vi "ModbusRdWrCam3.vi"() -> ()   [LabVIEW 2020]
uses:
  <vilib>/userdefined/High Color/IMAQdx.ctl
  <vilib>/Modbus/master/Create Master Instance (TCP).vi
  <vilib>/Modbus/master/Modbus Master.lvclass
  <vilib>/vision/driver/NI_Vision_Acquisition_Software.lvlib
panel:
  in  "Off/On":bool=TRUE
  out "Cam":bool
  in  "Session":T1="cam1"
  out "Image":T2(plugin-control)
  in  "5":i16(slide)=300 min=80 max=520 step=5 scale=80.0..520.0
  in  "4":i16(slide)=310 min=80 max=520 step=5 scale=80.0..520.0
  in  "3":i16(slide)=120 min=80 max=520 step=5 scale=80.0..520.0
  in  "2":i16(slide)=450 min=80 max=520 step=5 scale=80.0..520.0
  in  "1":i16(slide)=380 min=80 max=520 step=5 scale=80.0..520.0
  out "Modbus":bool
  in  "ip":string="192.168.4.1"
  out "Timer":u16=704
  in  "0":i16(slide)=285 min=80 max=520 step=5 scale=80.0..520.0
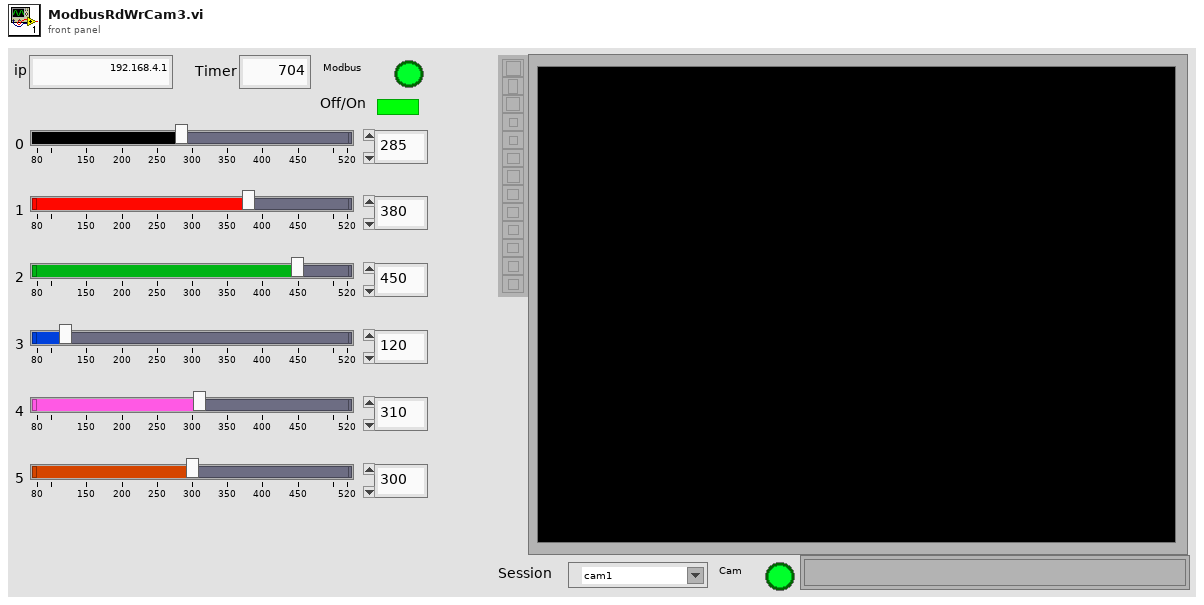
[diagram p1: front panel]
types:
  T1 = typedef "IMAQdx.ctl" = refnum<k21>
  T2 = typedef "IMAQ Image.ctl" = refnum<image>
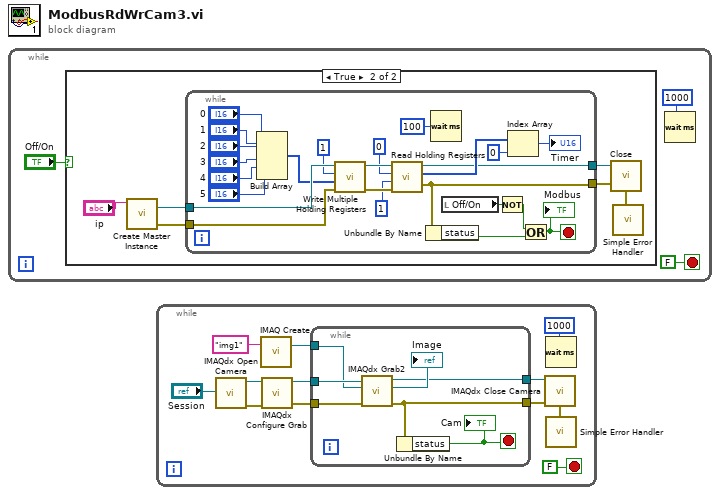
[diagram p0: block diagram]
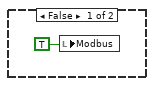
[diagram p2: hidden frame]
diagram:
  n1 = while {
    stop <- FALSE stop-if-true
    n2 = case shown="True" "Off/On" {
      frame False {
        n3 = local write "Modbus"(TRUE) -> ()
      }
      frame True {
        n4 = call-poly <vilib>:"Create Master Instance.vi"("address"="ip") -> ("error out"=w8:errorcluster, "TCP master instance"=w9:refnum<class "Modbus Master.lvclass">)  [unwired: 9 in]
        n5 = while {
          tunnel: w9 -> [w33]
          tunnel: w8 -> [w22]
          tunnel: [w14] -> w7
          tunnel: [w13] -> w6
          stop <- w16 stop-if-true
          n6 = Build Array("0", "1", "2", "3", "4", "5") -> (w32:i16[])
          n7 = call-dynamic "Write Multiple Holding Registers.vi"("error in (no error)"=w22, "holding register values"=w32, "starting address"=u16 1, "Modbus master in"=w33) -> ("error out"=w27:errorcluster, "Modbus master out"=w28:refnum<class "Modbus Master.lvclass">)  [unwired: 6 in]
          n8 = call-dynamic "Read Holding Registers.vi"("error in (no error)"=w27, "number of holding registers"=u16 1, "starting address"=u16 0, "Modbus master in"=w28) -> ("error out"=w13:errorcluster, "register values"=w24:u16[], "Modbus master out"=w14:refnum<class "Modbus Master.lvclass">)  [unwired: 5 in]
          n9 = Unbundle By Name(w13) -> ("status"=w15:bool)
          n10 = Wait (ms)(milliseconds to wait=u32 100) -> ()  [unwired: 1 out]
          n11 = local read "Off/On"() -> (w12:bool)
          n12 = Not(x=w12) -> (.not. x?=w11:bool)
          n13 = Index Array(array=w24, index=0) -> (element=→"Timer":u16)
          n14 = Or(x=w11, y=w15) -> (x .or. y?=w16:bool)
          "Modbus" <- w16
        }
        n15 = call-dynamic "Close.vi"("error in (no error)"=w6, "Modbus master in"=w7) -> ("error out"=w5:errorcluster)  [unwired: 9 in]
        n16 = call <vilib>:"Simple Error Handler.vi"("error in (no error)"=w5) -> ()  [unwired: 4 in, 5 out]
      }
    }
    n17 = Wait (ms)(milliseconds to wait=1000) -> ()  [unwired: 1 out]
  }
  n18 = while {
    stop <- FALSE stop-if-true
    n19 = call <vilib>:"IMAQdx Open Camera.vi"("Session In"="Session") -> ("error out"=w46:errorcluster, "Session Out"=w44:T1)  [unwired: 9 in]
    n20 = call "IMAQ Create"("Image Name"="img1") -> ("New Image"=w41:T2)  [unwired: 4 in, 1 out]
    n21 = call <vilib>:"IMAQdx Configure Grab.vi"("error in"=w46, "Session In"=w44) -> ("error out"=w45:errorcluster, "Session Out"=w43:T1)  [unwired: 8 in]
    n22 = while {
      tunnel: w45 -> [w53]
      tunnel: w43 -> [w52]
      tunnel: w41 -> [w50]
      tunnel: [w48] -> w37
      tunnel: [w47] -> w36
      stop <- w49 stop-if-true
      n23 = call <vilib>:"IMAQdx Grab2.vi"("error in"=w53, "Image In"=w50, "Session In"=w52) -> ("error out"=w47:errorcluster, "Image Out"=→"Image":T2, "Session Out"=w48:T1)  [unwired: 5 in, 1 out]
      n24 = Unbundle By Name(w47) -> ("status"=w49:bool)
      "Cam" <- w49
    }
    n25 = call <vilib>:"IMAQdx Close Camera.vi"("error in"=w36, "Session In"=w37) -> ("error out"=w35:errorcluster)  [unwired: 9 in]
    n26 = Wait (ms)(milliseconds to wait=1000) -> ()  [unwired: 1 out]
    n27 = call <vilib>:"Simple Error Handler.vi"("error in (no error)"=w35) -> ()  [unwired: 4 in, 5 out]
  }
